vi "PointerPosition.vi"(9 "Frame Properties (m)":T2, 10 "Reframed Position (m)":cluster{"x (m)":dbl, "y (m)":dbl, "z (m)":dbl} {"z (m)" format="%.1p"; "y (m)" format="%.1p"; "x (m)" format="%.1p"}) -> (1 "string":string, 2 "Position":T1)   [LabVIEW 2019]
uses:
  <vilib>/Utility/miscctls.llb/LVPositionTypeDef.ctl
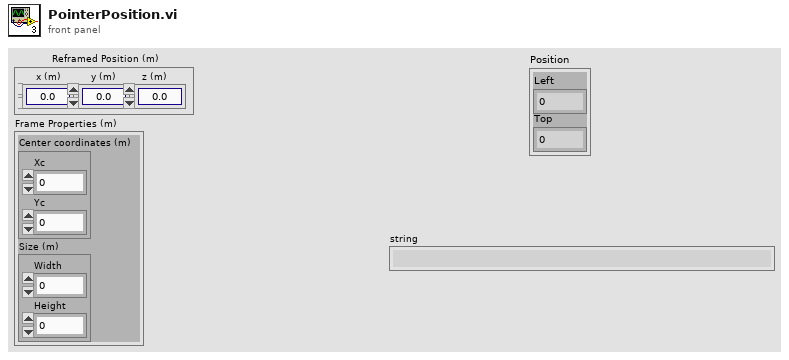
[diagram p1: front panel]
types:
  T1 = typedef "LVPositionTypeDef.ctl" = cluster{"Left":i32, "Top":i32}
  T2 = cluster{"Center coordinates (m)":cluster{"Xc":sgl, "Yc":sgl}, "Size (m)":cluster{"Width":sgl, "Height":sgl}}
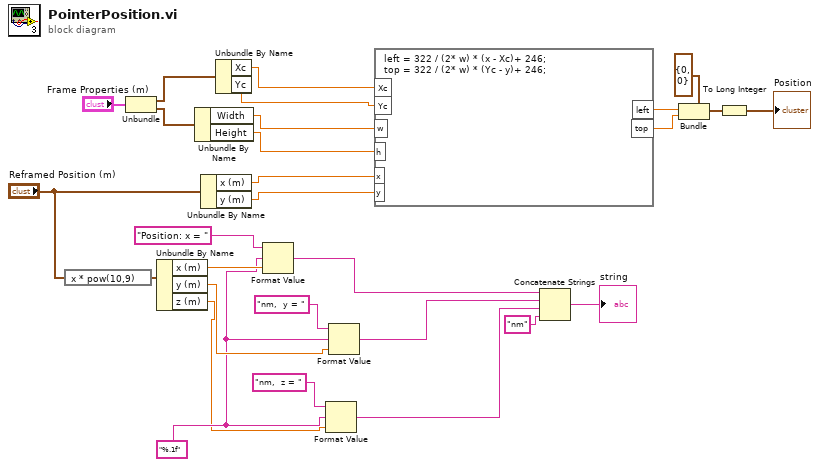
[diagram p0: block diagram]
diagram:
  w4 = "%.1f" ("format string")
  n1 = expression code="x * pow(10,9)"("Reframed Position (m)") -> (w11:cluster{"x (m)":dbl, "y (m)":dbl, "z (m)":dbl})
  n2 = Unbundle("Frame Properties (m)") -> ("Center coordinates (m)"=w27:cluster{"Xc":sgl, "Yc":sgl}, "Size (m)"=w26:cluster{"Width":sgl, "Height":sgl})
  n3 = Unbundle By Name(w11) -> ("x (m)"=w13:dbl, "y (m)"=w8:dbl, "z (m)"=w3:dbl)
  n4 = Unbundle By Name(w26) -> ("Width"=w21:sgl, "Height"=w20:sgl)
  n5 = Unbundle By Name("Reframed Position (m)") -> ("x (m)"=w25:dbl, "y (m)"=w24:dbl)
  n6 = Unbundle By Name(w27) -> ("Xc"=w23:sgl, "Yc"=w22:sgl)
  n7 = Format Value(string ("")="Position: x = " ("string"), format string=w4, value (0)=w13) -> (output string=w10:string)
  n8 = Format Value(string ("")="nm,  z = " ("string"), format string=w4, value (0)=w3) -> (output string=w2:string)
  n9 = Format Value(string ("")="nm,  y = " ("string"), format string=w4, value (0)=w8) -> (output string=w7:string)
  n10 = formula code="left = 322 / (2* w) * (x - Xc)+ 246;\ntop = 322 / (2* w) * (Yc - y)+ 246;"("Xc"=w23, "Yc"=w22, "w"=w21, "h"=w20, "x"=w25, "y"=w24) -> ("left"=w19:dbl, "top"=w18:dbl)
  n11 = Concatenate Strings(w10, w7, w2, "nm" ("string")) -> (→"string":string)
  n12 = Bundle(cluster=T1 {"Left"=0, "Top"=0} ("Position"), "Left"=w19, "Top"=w18) -> (w16:T1)
  n13 = To Long Integer(number=w16) -> (32bit integer=→"Position":T1)
